vi "Unpack 32I12's Packed into 24xI16 as 32xI16_Unaligned.vi"(5 "Skip Error Check":bool, 7 "Init?":bool, 8 "Error In":errorcluster, 11 "Input Array":i16[](array[numeric])) -> (0 "Error Out":errorcluster, 3 "Output Array":i16[](array[numeric]))   [LabVIEW 2012]
uses:
  <vilib>/Utility/tdmsutil.llb/TDMS Generate Random Data (I16).vi
  <userlib>/FlexRIO Host Library/FlexRIO Host API/Packer and Unpacker/32ch 12-bit Pack/Test Bench/ProcessingDLL/Release/ProcessingDLL.dll
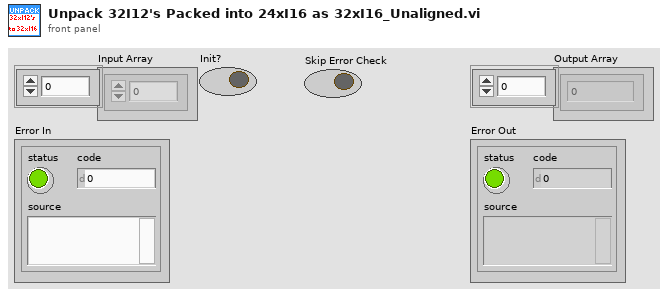
[diagram p1: front panel]
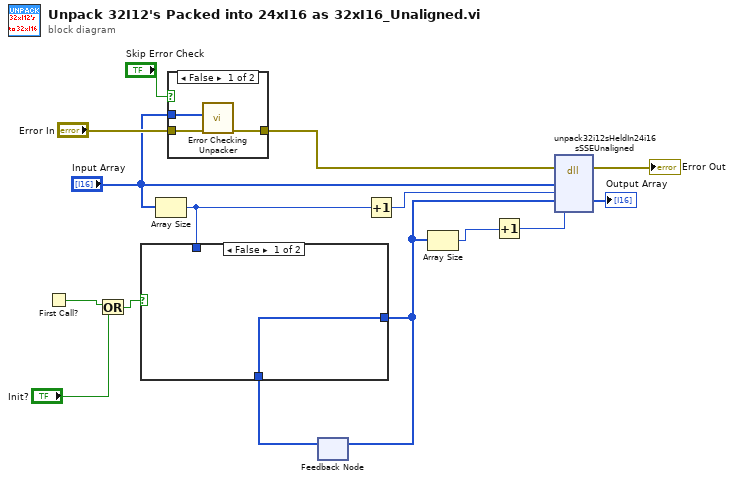
[diagram p0: block diagram]
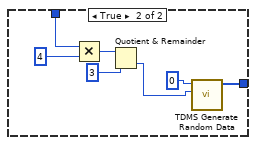
[diagram p3: hidden frame]
diagram:
  n1 = First Call?() -> (First Call?: T/F=w2:bool)
  n2 = Or(x=w2, y="Init?") -> (x .or. y?=w3:bool)
  n3 = Array Size(array="Input Array") -> (size(s)=w13:i32)
  n4 = case shown="False" "Skip Error Check" {
    tunnel: "Error In" -> [w18 w19]
    tunnel: "Input Array" -> [w17 _]
    tunnel: [w16 w19] -> w5
    frame False {
      n5 = call <userlib>:"Error Checking Unpacker.vi"("error in"=w18, "packed i12s"=w17) -> ("error out"=w16:errorcluster)  [unwired: 9 in]
    }
    frame True {
    }
  }
  n6 = feedback #1() -> (w9:i16[])  [unwired: 1 in]
  n7 = case shown="False" w3 {
    tunnel: w13 -> [_ w26]
    tunnel: [w20 w21] -> w10
    tunnel: w9 -> [w20 _]
    frame False {
    }
    frame True {
      n8 = Multiply(x=w26, y=4) -> (x*y=w24:i32)
      n9 = Quotient & Remainder(x=w24, y=3) -> (floor(x/y)=w22:i32)  [unwired: 1 out]
      n10 = call-poly <vilib>:"TDMS Generate Random Data.vi"("number of samples"=w22, "data type"=i16 0) -> ("data"=w21:i16[])  [unwired: 8 in, 1 out]
    }
  }
  n11 = feedback-in #1(w10) -> ()
  n12 = Increment(x=w13) -> (x+1=w15:i32)
  n13 = Array Size(array=w10) -> (size(s)=w12:i32)
  n14 = Increment(x=w12) -> (x+1=w14:i32)
  n15 = dll-call lib="C:/Program Files (x86)/National Instruments/LabVIEW 2012/user.lib/FlexRIO Host Library/FlexRIO Host API/Packer and Unpacker/32ch 12-bit Pack/Test Bench/ProcessingDLL/Release/ProcessingDLL.dll" fn="unpack32i12sHeldIn24i16sSSEUnaligned"(error in=w5, "source"="Input Array", "sourceSize"=w15, "destination"=w10, "destinationSize"=w14) -> (error out=→"Error Out":errorcluster, "destination"=→"Output Array":i16[])  [unwired: 6 in, 1 out]
